vi "Compare Strings.vi"(1 "y":string, 2 "x":string) -> (0 "Equal?":bool)   [LabVIEW 2016, in "SLL String.lvlib"]
doc: "Compares two strings ignoring whitespaces at ends and case sensitivity."
uses:
  SLL String.lvlib
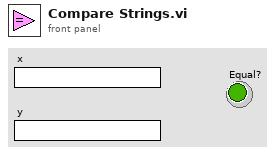
[diagram p1: front panel]
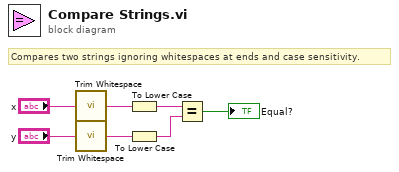
[diagram p0: block diagram]
diagram:
  # "Compares two strings ignoring whitespaces at ends and case sensitivity."
  n1 = call <vilib>:"Trim Whitespace.vi"("string"="x") -> ("trimmed string"=w4:string)  [unwired: 1 in]
  n2 = call <vilib>:"Trim Whitespace.vi"("string"="y") -> ("trimmed string"=w3:string)  [unwired: 1 in]
  n3 = To Lower Case(string=w4) -> (all lower case string=w2:string)
  n4 = To Lower Case(string=w3) -> (all lower case string=w1:string)
  n5 = Equal?(x=w2, y=w1) -> (x = y?=→"Equal?":bool)
